vi "_utils_ Remove Timeout Error.vi"(0 "error in":errorcluster) -> (1 "Operation timed out?":bool, 2 "error out":errorcluster)   [LabVIEW 2014]
doc: "Reports wether the input error cluster shows that a Timeout error occured, and replaces it with a No Error cluster structure."
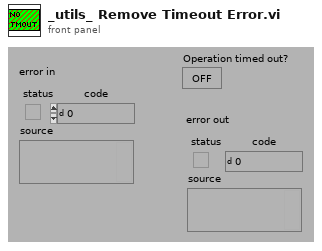
[diagram p1: front panel]
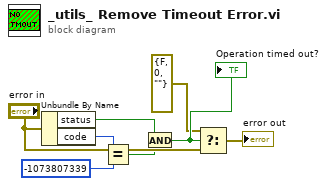
[diagram p0: block diagram]
diagram:
  n1 = Unbundle By Name("error in") -> ("status"=w7:bool, "code"=w1:i32)
  n2 = Equal?(x=w1, y=-1073807339) -> (x = y?=w3:bool)
  n3 = And(x=w7, y=w3) -> (x .and. y?=w8:bool)
  "Operation timed out?" <- w8
  n4 = Select(t=errorcluster {"status"=FALSE, "code"=0, "source"=""}, s=w8, f="error in") -> (s? t:f=→"error out":errorcluster)
